vi "Create mask array.vi"(8 "Left error in":errorcluster, 11 "Right Error in":errorcluster) -> (0 "Left error out":errorcluster, 3 "Right error out":errorcluster, 4 "Left Cam Masks":T1[](array[typedef]), 5 "Right Cam Masks":T1[](array[typedef]))   [LabVIEW 2009]
uses:
  <vilib>/vision/Image Controls.llb/IMAQ Image.ctl
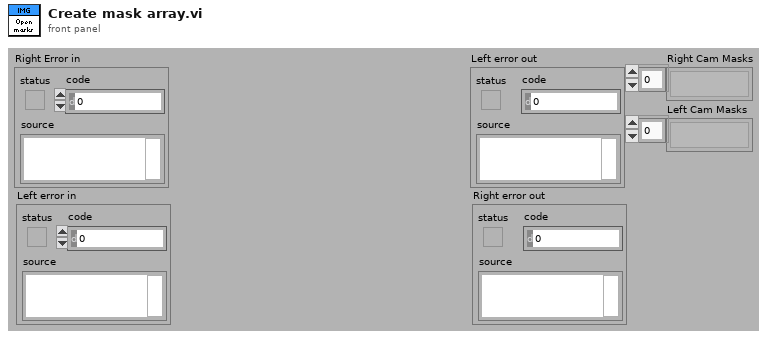
[diagram p1: front panel]
types:
  T1 = typedef "IMAQ Image.ctl" = refnum<image>
  T2 = typedef "Image Type" = u32
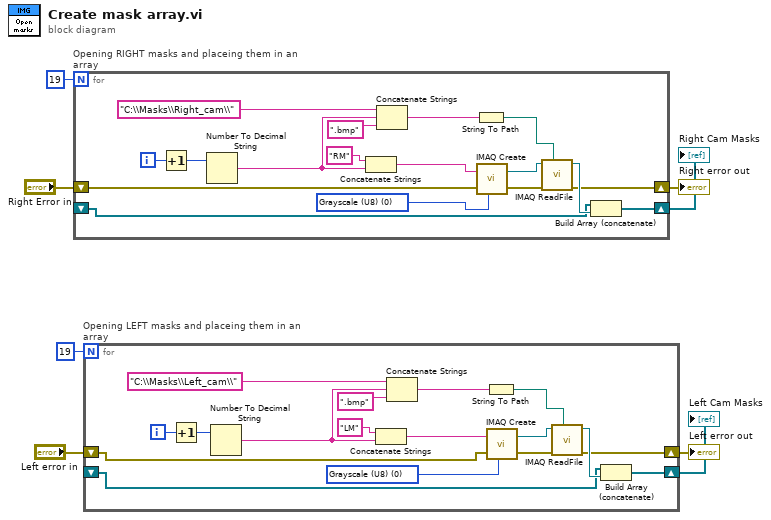
[diagram p0: block diagram]
diagram:
  n1 = for "Opening RIGHT masks and placeing them in an array" {
    N: 19 -> [_]
    shift-right: [w19] -> w2
    shift-left: _ -> [w18]
    shift-right: [w17] -> w3
    shift-left: "Right Error in" -> [w16]
    i -> [w23]
    w21 = T2 0 items=["Grayscale (U8)", "Grayscale (I16)", "Grayscale (SGL)", "Complex (CSG)", "RGB (U32)", "HSL (U32)", "RGB (U64)", "Grayscale (U16)"] ("Image Type")
    n2 = Increment(x=w23) -> (x+1=w22:i32)
    n3 = Number To Decimal String(number=w22) -> (decimal integer string=w10:string)  [unwired: 1 in]
    n4 = Concatenate Strings("RM" ("element"), w10) -> (w9:string)
    n5 = Concatenate Strings("C:\\Masks\\Right_cam\\", w10, ".bmp") -> (w11:string)
    n6 = String To Path(string=w11) -> (path=w12:path)
    n7 = call "IMAQ Create"("Image Name"=w9, "Image Type"=w21, "error in (no error)"=w16) -> ("New Image"=w24:T1, "error out"=w25:errorcluster)  [unwired: 2 in]
    n8 = call "IMAQ ReadFile"("File Path"=w12, "error in (no error)"=w25, "Image"=w24) -> ("error out"=w17:errorcluster, "Image Out"=w20:T1)  [unwired: 4 in, 3 out]
    n9 = Build Array (concatenate)(w18, w20) -> (w19:T1[])
  }
  "Right error out" <- w3
  "Right Cam Masks" <- w2
  n10 = for "Opening LEFT masks and placeing them in an array" {
    N: 19 -> [_]
    shift-right: [w36] -> w1
    shift-left: _ -> [w35]
    shift-right: [w34] -> w4
    shift-left: "Left error in" -> [w33]
    i -> [w40]
    w38 = T2 0 items=["Grayscale (U8)", "Grayscale (I16)", "Grayscale (SGL)", "Complex (CSG)", "RGB (U32)", "HSL (U32)", "RGB (U64)", "Grayscale (U16)"] ("Image Type")
    n11 = Increment(x=w40) -> (x+1=w39:i32)
    n12 = Number To Decimal String(number=w39) -> (decimal integer string=w27:string)  [unwired: 1 in]
    n13 = Concatenate Strings("LM" ("element"), w27) -> (w26:string)
    n14 = Concatenate Strings("C:\\Masks\\Left_cam\\", w27, ".bmp") -> (w28:string)
    n15 = String To Path(string=w28) -> (path=w29:path)
    n16 = call "IMAQ Create"("Image Name"=w26, "Image Type"=w38, "error in (no error)"=w33) -> ("New Image"=w41:T1, "error out"=w42:errorcluster)  [unwired: 2 in]
    n17 = call "IMAQ ReadFile"("File Path"=w29, "error in (no error)"=w42, "Image"=w41) -> ("error out"=w34:errorcluster, "Image Out"=w37:T1)  [unwired: 4 in, 3 out]
    n18 = Build Array (concatenate)(w35, w37) -> (w36:T1[])
  }
  "Left error out" <- w4
  "Left Cam Masks" <- w1
